vi "Get Wheel Property by Name.vi"(7 "wheel index":i32, 8 "error in (no error)":errorcluster, 10 "parameter name":string, 11 "steering frame reference in":refnum<data-value>) -> (0 "error out":errorcluster, 1 "found?":bool, 2 "parameter value":variant, 3 "steering frame reference out":refnum<data-value>)   [LabVIEW 2017, in "NI_Robotics_Configure Steering Frame.lvlib"]
uses:
  <vilib>/robotics/Dialog/Configure Steering Frame/NI_Robotics_Configure Steering Frame.lvlib
  <vilib>/robotics/Steering/Steering Frame/NI_Robotics_Steering Frame.lvclass
  <vilib>/robotics/Steering/Steering Frame/NI_Robotics_Steering Frame.lvclass/NI_Robotics_Steering Frame.ctl
  <vilib>/robotics/Steering/Steering Frame/Get Multiple Wheels in Steering Frame.vi
  <vilib>/robotics/Steering/Wheel/NI_Robotics_Wheel.lvclass
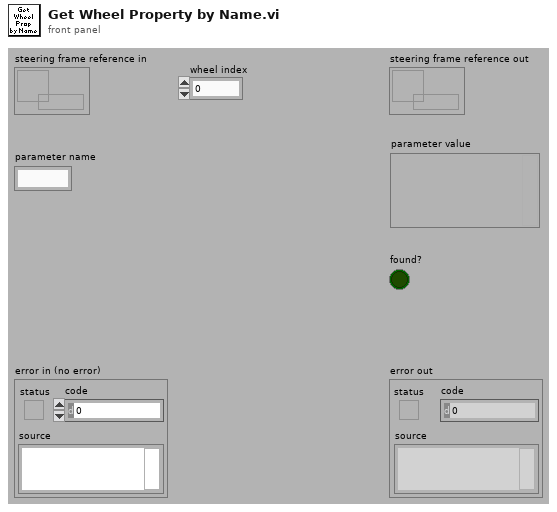
[diagram p1: front panel]
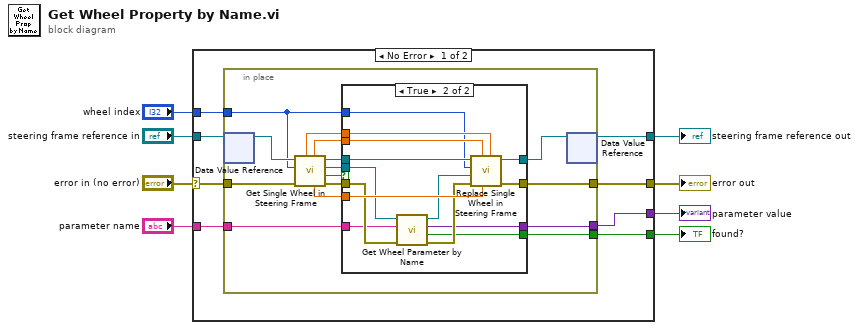
[diagram p0: block diagram]
diagram:
  n1 = case shown="No Error" "error in (no error)" {
    selector: "error in (no error)" -> [w13 w49]
    tunnel: [w9 w49] -> w7
    tunnel: "steering frame reference in" -> [w14 w48]
    tunnel: [w10 w48] -> w5
    tunnel: "wheel index" -> [w16 _]
    tunnel: "parameter name" -> [w15 _]
    tunnel: [w11 _] -> w2
    tunnel: [w12 _] -> w1
    frame No Error {
      n2 = in-place {
        in-place-border: w16 -> [w21]
        in-place-border: w15 -> [w31]
        in-place-border: w13 -> [w26]
        in-place-border: [w30] -> w11
        in-place-border: [w19] -> w9
        in-place-border: [w17] -> w12
        n3 = in-place-dvr #1(w14) -> (w29:refnum<class "NI_Robotics_Steering Frame.lvclass">)  [unwired: 1 out]
        n4 = call <vilib>:"Get Single Wheel in Steering Frame.vi"("error in (no error)"=w26, "wheel index"=w21, "steering frame in"=w29) -> ("error out"=w27:errorcluster, "found?"=w18:bool, "wheel"=w28:refnum<class "NI_Robotics_Wheel.lvclass">, "steering frame out"=w25:refnum<class "NI_Robotics_Steering Frame.lvclass">, "frame angle (rad)"=w22:dbl, "y position"=w24:dbl, "x position"=w23:dbl)  [unwired: 2 in]
        n5 = case shown="True" w18 {
          tunnel: w31 -> [_ w37]
          tunnel: [_ w35] -> w30
          tunnel: w28 -> [_ w40]
          tunnel: w27 -> [w32 w38]
          tunnel: w25 -> [w33 w47]
          tunnel: w24 -> [_ w46]
          tunnel: w23 -> [_ w45]
          tunnel: w22 -> [_ w44]
          tunnel: w21 -> [_ w43]
          tunnel: [w33 w42] -> w20
          tunnel: [w32 w41] -> w19
          tunnel: [_ w34] -> w17
          frame False {
          }
          frame True {
            n6 = call-dynamic "Get Wheel Parameter by Name.vi"("error in (no error)"=w38, "parameter name"=w37, "wheel in"=w40) -> ("error out"=w36:errorcluster, "found?"=w35:bool, "parameter value"=w34:variant, "wheel out"=w39:refnum<class "NI_Robotics_Wheel.lvclass">)  [unwired: 5 in]
            n7 = call <vilib>:"Replace Single Wheel in Steering Frame.vi"("x position"=w45, "frame angle (rad)"=w44, "y position"=w46, "error in (no error)"=w36, "wheel"=w39, "wheel index"=w43, "steering frame in"=w47) -> ("error out"=w41:errorcluster, "steering frame out"=w42:refnum<class "NI_Robotics_Steering Frame.lvclass">)  [unwired: 2 in, 1 out]
          }
        }
        n8 = in-place-dvr #1(w20) -> (w10:refnum<data-value>)  [unwired: 1 out]
      }
    }
    frame Error {
    }
  }
  "error out" <- w7
  "steering frame reference out" <- w5
  "parameter value" <- w1
  "found?" <- w2
